vi "Initialize Event References.vi"(8 "error in (no error)":errorcluster) -> (0 "error out":errorcluster, 3 "Event-References":T1)   [LabVIEW 2018, in "Actor.lvclass"]
uses:
  Actor.lvclass
  Event-References.ctl
  Stop.ctl
  Actor Class Launched.ctl
  Example-Request.ctl
  Example-Reply.ctl
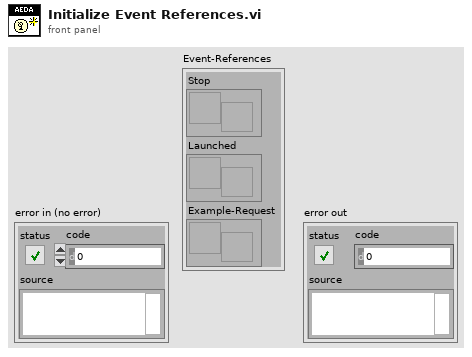
[diagram p1: front panel]
types:
  T1 = typedef "Actor.lvclass/Event-References.ctl" = cluster{"Stop":refnum<user-event>, "Launched":refnum<user-event>, "Example-Request":refnum<user-event>}
  T2 = typedef "Actor.lvclass/Example-Request.ctl" = cluster{"Number":bool, "String":string}
  T3 = typedef "Actor.lvclass/Actor Class Launched.ctl" = cluster{"Launched State":refnum<class "Actor.lvclass">}
  T4 = typedef "Actor.lvclass/Stop.ctl" = enum16{"Normal", "Emergency"}
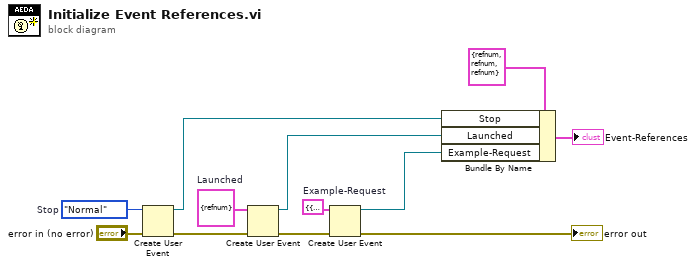
[diagram p0: block diagram]
diagram:
  w3 = cluster{"Number":T2, "Reply":refnum<user-event>} {"Number"={"Number"=FALSE, "String"=""}, "Reply"=refnum}  # Example-Request
  w11 = T3 {"Launched State"=refnum}  # Launched
  w10 = Stop."Normal"  # Stop
  n1 = Create User Event(user event datatype=w10, error in="error in (no error)") -> (user event=w7:refnum<user-event>, error out=w12:errorcluster)
  n2 = Create User Event(user event datatype=w11, error in=w12) -> (user event=w6:refnum<user-event>, error out=w4:errorcluster)
  n3 = Create User Event(user event datatype=w3, error in=w4) -> (user event=w2:refnum<user-event>, error out=→"error out":errorcluster)
  n4 = Bundle By Name(cluster=T1 {"Stop"=refnum, "Launched"=refnum, "Example-Request"=refnum} ("Actor-Events"), "Stop"=w7, "Launched"=w6, "Example-Request"=w2) -> (→"Event-References":T1)
